vi "Set PDOs mapping )setting(.vi"() -> ()   [LabVIEW 2016]
uses:
  <vilib>/CANopenLib/CANOPEN.llb/CANopen SDO Create.vi
  Set PDOs mapping.vi
  <vilib>/CANopenLib/CANOPEN.llb/CANopen SDO Close.vi
  <vilib>/CANopenLib/CANOPEN.llb/CANopen Interface Close.vi
panel:
  out "error out":errorcluster
  out "completion codes":u32[](array[numeric])
  in  "Motor":u8(ring) items=["Right", "Left"]
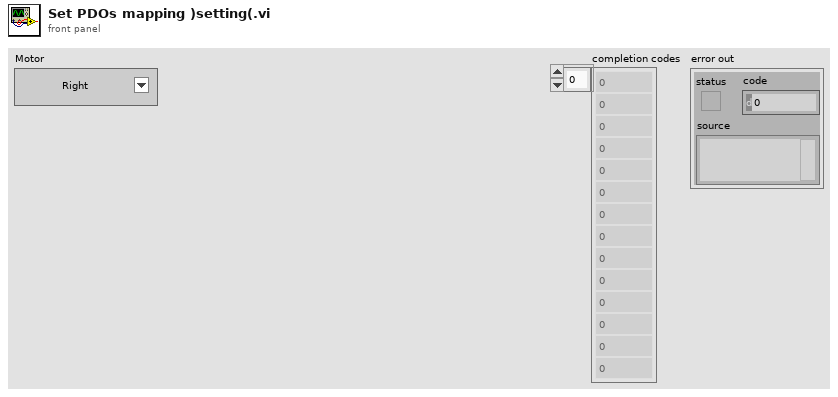
[diagram p1: front panel]
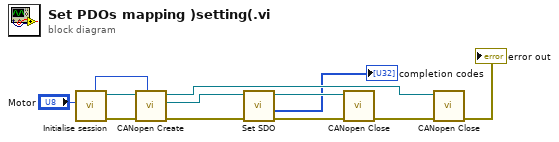
[diagram p0: block diagram]
diagram:
  n1 = call "Initialise session.vi"("Motor"="Motor") -> ("error out"=w8:errorcluster, "interface object out"=w12:refnum<k20>, "Used Node ID"=w7:u8)  [unwired: 8 in]
  n2 = call-poly <vilib>:"CANopen Create.vi"("node-ID"=w7, "error in (no error)"=w8, "interface object in"=w12) -> ("error out"=w9:errorcluster, "SDO object out"=w11:refnum<k20>, "interface object out"=w10:refnum<k20>)  [unwired: 6 in]
  n3 = call-poly "Set SDO.vi"("error in (no error)"=w9, "SDO object in"=w11) -> ("error out"=w5:errorcluster, "completion codes"=→"completion codes":u32[], "SDO object out"=w4:refnum<k20>)  [unwired: 7 in]
  n4 = call-poly <vilib>:"CANopen Close.vi"("error in (no error)"=w5, "SDO object in"=w4) -> ("error out"=w6:errorcluster)  [unwired: 9 in]
  n5 = call-poly <vilib>:"CANopen Close.vi"("error in (no error)"=w6, "interface object in"=w10) -> ("error out"=→"error out":errorcluster)  [unwired: 9 in]
